vi "Pause Process.vi"(8 "error in (no error)":errorcluster, 11 "iProcess Model in":refnum<class "iProcess Model.lvclass">) -> (0 "error out":errorcluster, 3 "iProcess Model out":refnum<class "iProcess Model.lvclass">)   [LabVIEW 2019, in "iProcess Model.lvclass"]
uses:
  <vilib>/gpm_packages/@cs/Car-wash/Source/iProcess Model/iProcess Model/iProcess Model.lvclass
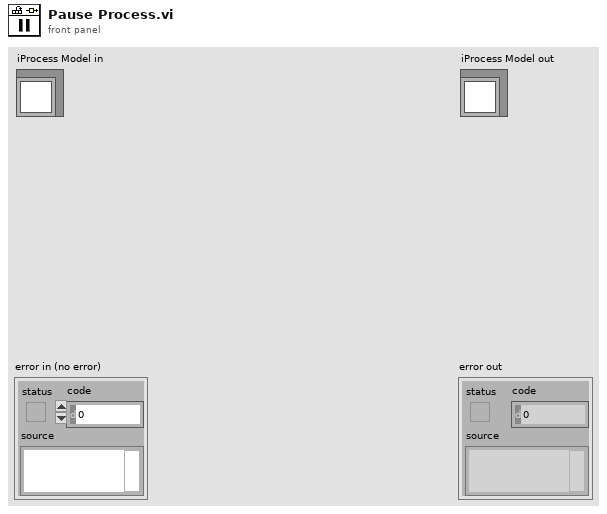
[diagram p1: front panel]
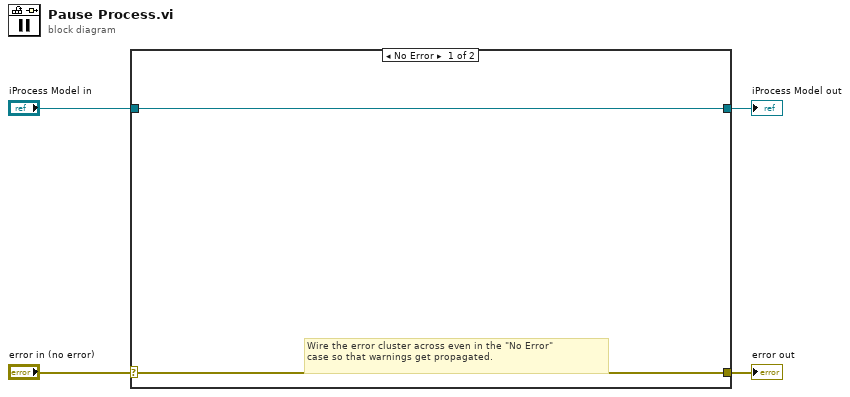
[diagram p0: block diagram]
diagram:
  n1 = case shown="No Error" "error in (no error)" {
    selector: "error in (no error)" -> [w5 w8]
    tunnel: [w5 w8] -> w3
    tunnel: [w6 w7] -> w1
    tunnel: "iProcess Model in" -> [w6 w7]
    frame No Error {
      # "Wire the error cluster across even in the \"No Error\"\ncase so that warnings get propagated."
    }
    frame Error {
    }
  }
  "error out" <- w3
  "iProcess Model out" <- w1
